vi "Read Example With Events (advanced).vi"(0 "Source Address":u8=228 format="%.0x", 2 "Device Selected":i32, 11 "Error In":errorcluster) -> (15 "Error Out":errorcluster)   [LabVIEW 2014, in "GEA2_Toolkit.lvlib"]
doc: "This event driven standalone VI continuously monitors the GEA bus and parses messages as they appear."
uses:
  library/GEA2_Toolkit.lvlib
  type defs/Data Out.ctl
  Washer HCC/Washer HCC NEWFI/LabVIEW GEA2 Toolkit/LabVIEW_GEA2_Toolkit.lvlibp
panel:
  out "Data Out":T1[](array[typedef]) {"CRC" format="%04x"; "Length" format="%02x"; "Command" format="%02x"; "Destination" format="%02x"; "Source" format="%02x"}
  in  "Stop":bool
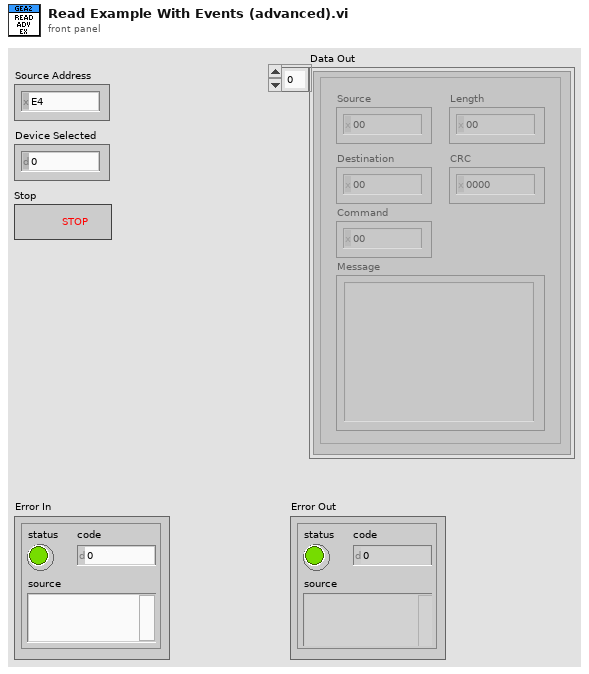
[diagram p1: front panel]
types:
  T1 = typedef "GEA2_Toolkit.lvlib/Data Out.ctl" = cluster{"Source":u8, "Destination":u8, "Command":u8, "Length":u8, "CRC":u16, "Message":string}
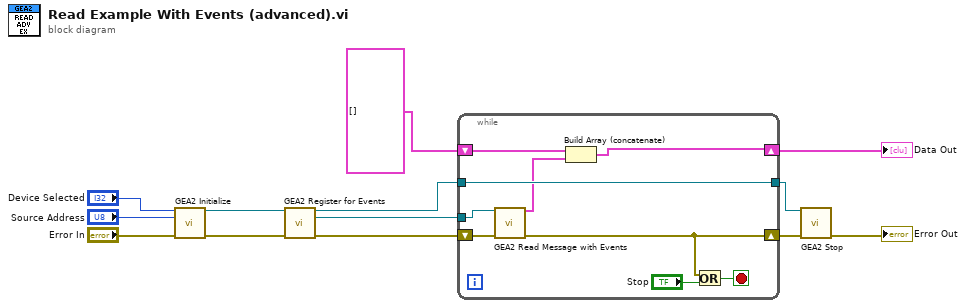
[diagram p0: block diagram]
diagram:
  n1 = call "GEA2 Initialize.vi"("Board Index"="Device Selected", "Source Address"="Source Address", "error in"="Error In") -> ("GEA2 Reference Out"=w1:refnum<k24>, "error out"=w11:errorcluster)  [unwired: 10 in, 1 out]
  n2 = call "GEA2 Register for Events.vi"("GEA2 Reference In"=w1, "Error In"=w11) -> ("GEA2 Reference Out"=w7:refnum<k24>, "GEA2 Event Registration"=w2:refnum<event-registration>, "Error Out"=w10:errorcluster)  [unwired: 11 in]
  n3 = while {
    tunnel: w2 -> [w22]
    tunnel: [w19] -> w8
    tunnel: w7 -> [w19]
    shift-right: [w17] -> w9
    shift-left: w10 -> [w18]
    shift-right: [w15] -> w6
    shift-left: T1[] [] -> [w14]
    stop <- w20 stop-if-true
    n4 = call "GEA2 Read Message with Events.vi"("GEA2 Event Registration"=w22, "Error In"=w18) -> ("Coverted Data Out"=w16:T1, "Error Out"=w17:errorcluster)  [unwired: 12 in]
    n5 = Build Array (concatenate)(w14, w16) -> (w15:T1[])
    n6 = Or(x=w17, y="Stop") -> (x .or. y?=w20:bool)
  }
  "Data Out" <- w6
  n7 = call "GEA2 Stop.vi"("GEA2 Reference In"=w8, "Error In"=w9) -> ("Error Out"=→"Error Out":errorcluster)  [unwired: 13 in]
